vi "Cron TimeUnitNextJob.vi"(10 "Next Occurence":timestamp) -> (2 "next event (ms)":i32)   [LabVIEW 2013, in "openCron.lvlib"]
uses:
  openCron.lvlib
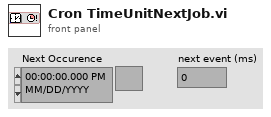
[diagram p1: front panel]
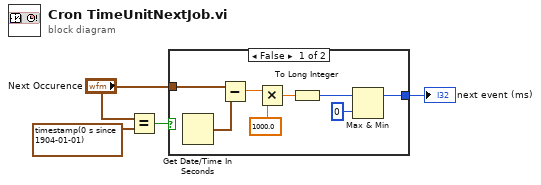
[diagram p0: block diagram]
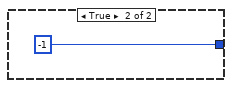
[diagram p2: hidden frame]
diagram:
  n1 = Equal?(x="Next Occurence", y=timestamp(0 s since 1904-01-01)) -> (x = y?=w1:bool)
  n2 = case shown="False" w1 {
    tunnel: [w5 -1] -> w4
    tunnel: "Next Occurence" -> [w11 _]
    frame False {
      n3 = Get Date/Time In Seconds() -> (seconds since 1Jan1904=w12:timestamp)
      n4 = Subtract(x=w11, y=w12) -> (x-y=w10:dbl)
      n5 = Multiply(x=w10, y=1000.0) -> (x*y=w8:dbl)
      n6 = To Long Integer(number=w8) -> (32bit integer=w6:i32)
      n7 = Max & Min(x=w6, y=0) -> (max(x,y)=w5:i32)  [unwired: 1 out]
    }
    frame True {
    }
  }
  "next event (ms)" <- w4
